vi "Find Available Project Name.vi"(8 "error in (no error)":errorcluster, 10 "Project folder":path, 11 "Project name":string="Untitled Project") -> (0 "error out":errorcluster, 2 "Project folder out":path, 3 "Project name out":string)   [LabVIEW 2021]
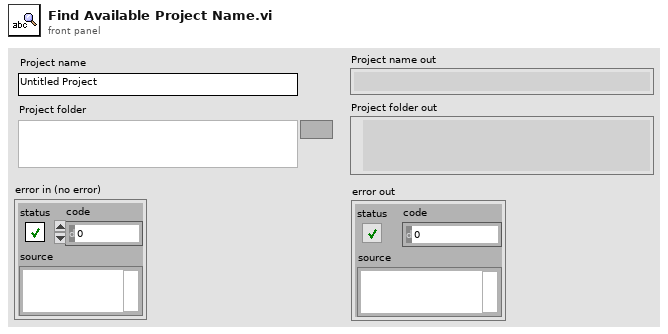
[diagram p1: front panel]
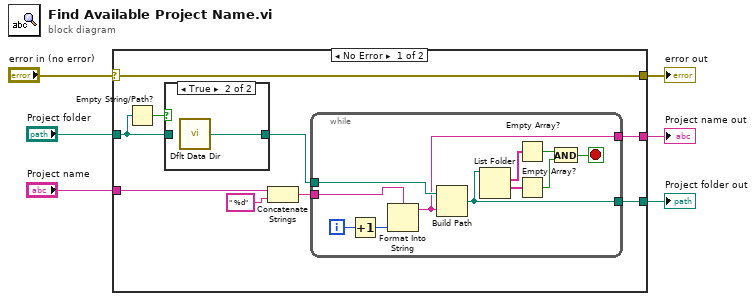
[diagram p0: block diagram]
diagram:
  n1 = case shown="No Error" "error in (no error)" {
    selector: "error in (no error)" -> [w12 w29]
    tunnel: "Project folder" -> [w14 _]
    tunnel: "Project name" -> [w9 _]
    tunnel: [w12 w29] -> w1
    tunnel: [w11 _] -> w3
    tunnel: [w10 _] -> w2
    frame No Error {
      n2 = Empty String/Path?(string/path=w14) -> (empty?=w15:bool)
      n3 = case shown="True" w15 {
        tunnel: [w27 w28] -> w13
        tunnel: w14 -> [w27 _]
        frame False {
        }
        frame True {
          n4 = call <vilib>:"Dflt Data Dir.vi"() -> ("App:Default Data Directory"=w28:path)
        }
      }
      n5 = Concatenate Strings(w9, " %d" ("string")) -> (w7:string)
      n6 = while {
        tunnel: w13 -> [w26]
        tunnel: w7 -> [w25]
        tunnel: [w18] -> w11
        tunnel: [w17] -> w10
        i -> [w24]
        stop <- w16 stop-if-true
        n7 = Increment(x=w24) -> (x+1=w23:i32)
        n8 = Format Into String(format string=w25, w23) -> (resulting string=w18:string)  [unwired: 2 in, 1 out]
        n9 = Build Path(base path=w26, name or relative path=w18) -> (appended path=w17:path)
        n10 = List Folder(path=w17) -> (filenames=w22:string[], folder names=w21:string[])  [unwired: 3 in, 2 out]
        n11 = Empty Array?(array=w22) -> (empty?=w20:bool)
        n12 = Empty Array?(array=w21) -> (empty?=w19:bool)
        n13 = And(x=w20, y=w19) -> (x .and. y?=w16:bool)
      }
    }
    frame Error {
    }
  }
  "Project folder out" <- w2
  "Project name out" <- w3
  "error out" <- w1
